vi "Angle to Ticks.vi"(8 "error in (no error)":errorcluster, 10 "angle (radian)":dbl, 11 "KUKA youBot arm motor_EtherCAT in":refnum<class "NI_Robotics_KUKA youBot Arm Motor_EtherCAT.lvclass">) -> (0 "error out":errorcluster, 2 "ticks":i32=1, 3 "KUKA youBot arm motor_EtherCAT out":refnum<class "NI_Robotics_KUKA youBot Arm Motor_EtherCAT.lvclass">)   [LabVIEW 2017, in "NI_Robotics_KUKA youBot Host.lvlib" / "NI_Robotics_KUKA youBot Arm Motor_EtherCAT.lvclass"]
uses:
  <vilib>/robotics/KUKA youBot/Motor/Arm Motor EtherCAT/NI_Robotics_KUKA youBot Arm Motor_EtherCAT.lvclass
  <vilib>/robotics/KUKA youBot/Motor/Arm Motor EtherCAT/NI_Robotics_KUKA youBot Arm Motor_EtherCAT.lvclass/NI_Robotics_KUKA youBot Arm Motor_EtherCAT.ctl
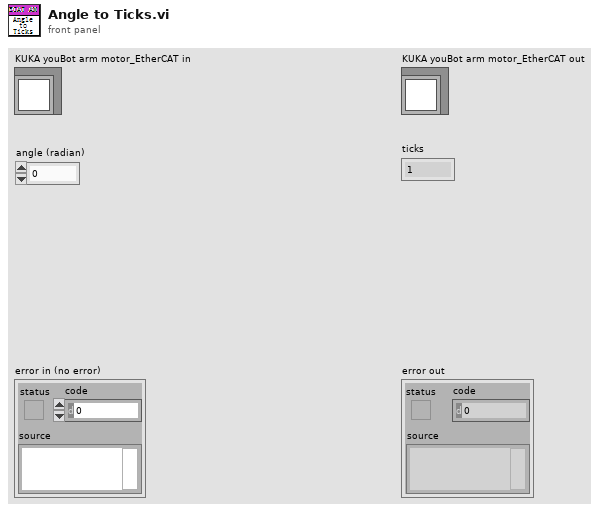
[diagram p1: front panel]
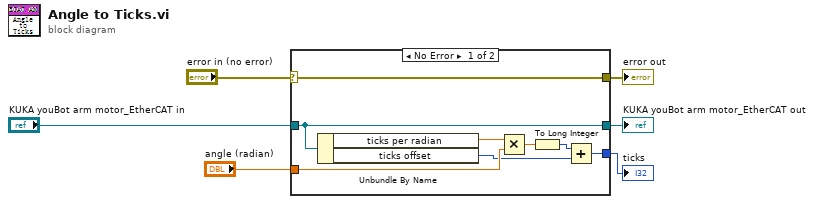
[diagram p0: block diagram]
diagram:
  n1 = case shown="No Error" "error in (no error)" {
    selector: "error in (no error)" -> [w14 w15]
    tunnel: [w14 w15] -> w5
    tunnel: [w13 w16] -> w3
    tunnel: "KUKA youBot arm motor_EtherCAT in" -> [w13 w16]
    tunnel: "angle (radian)" -> [w9 _]
    tunnel: [w7 _] -> w1
    frame No Error {
      n2 = Unbundle By Name(w13) -> ("ticks per radian"=w10:dbl, "ticks offset"=w8:i32)
      n3 = Multiply(x=w10, y=w9) -> (x*y=w12:dbl)
      n4 = To Long Integer(number=w12) -> (32bit integer=w11:i32)
      n5 = Add(x=w11, y=w8) -> (x+y=w7:i32)
    }
    frame Error {
    }
  }
  "error out" <- w5
  "KUKA youBot arm motor_EtherCAT out" <- w3
  "ticks" <- w1
